vi "6 Cyl Diesel with 1 VR Crank + 2 Hall Cams + Knock.vi"() -> ()   [LabVIEW 2013]
uses:
  Version Token.ctl
  APU/Settings.ctl
  APU/Input.ctl
  APU/Output.ctl
  Analog Replay/Settings.ctl
  Analog Replay/Input.ctl
  Analog Replay/Load Input.ctl
  Digital Pattern Generation/Load Input.ctl
  Digital Pattern Generation/Settings.ctl
  Digital Pattern Generation/Input.ctl
  ECU Event/Timing/Measure Output.ctl
  ECU Event/Timing/Measure Settings.ctl
  ECU Event/Timing/Capture Output.ctl
  Knock Sensor/Generate Input.ctl
  Knock Sensor/Cylinder Input.ctl
  Knock Sensor/Cylinder Settings.ctl
  Knock Sensor/Generate Settings.ctl
  APU/Shared Settings.ctl
  <vilib>/Platform/TimedLoop/XDataNode/timing_clust.ctl
  <vilib>/Platform/TimedLoop/XDataNode/nitl_modes.ctl
  <vilib>/Platform/TimedLoop/XDataNode/wakeup.ctl
  ECU Event/Timing/Capture Settings.ctl
  <vilib>/rvi/DataTransferAndStorage/Container/Common/niFpgaContainerGetUniqueNameForEmu.vi
  <vilib>/rvi/DataTransferAndStorage/Container/Common/niFpgaContainerSetEmuInfo.vi
  <vilib>/rvi/eio/common/nirviEmuReportErrorAndStop.vi
  <vilib>/rvi/Emulation/niFpgaSctlEmulationGetInTimedLoop.vi
  <vilib>/rvi/Emulation/niFpgaEmulationReportErrorSimple.vi
  <vilib>/rvi/Emulation/niFpgaGetClockAttributes.vi
  <vilib>/rvi/Emulation/niFpgaCriticalErrorInLSC.vi
  <vilib>/rvi/eio/common/nirviEmuTemplateMethod_errors.vi
  ECU Event/Timing/Measure Events (40MHz).vi
  <vilib>/Platform/TimedLoop/XDataNode/XDataNode.xnode
  <vilib>/rvi/LocalResourceManager/LocalResourceManager.xnode
  <vilib>/eio/EIONode/EIONode.xnode
  <vilib>/Platform/TimedLoop/XDataNode/XDNodeRunTimeDep.lvlib
  APU/APU.lvlib
  Analog Replay/Analog Replay.lvlib
  Digital Pattern Generation/Digital Pattern Generation.lvlib
  ECU Event/Timing/ECU Event Timing.lvlib
  Knock Sensor/Knock Sensor.lvlib
  Engine Simulation Toolkit.lvlib
panel:
  in  "shared settings.apu 1":T1 {"cycle start" format="%#.15g"}
  in  "go.apu 1":bool
  in  "settings.Knock AO 2.Cylinder 5":T2
  in  "settings.Knock AO 2.Cylinder 6":T2
  in  "input.Knock AO 2.Cylinder 5":T3={"probability compare"=65535, "high freq scaler"=0.0, "trigger position"=0}
  in  "input.Knock AO 2.Cylinder 6":T3={"probability compare"=65535, "high freq scaler"=0.0, "trigger position"=0}
  in  "settings.Knock AO 2":T4
  in  "settings.Knock AO 2.Cylinder 1":T2
  in  "settings.Knock AO 2.Cylinder 2":T2
  in  "settings.Knock AO 2.Cylinder 3":T2
  in  "settings.Knock AO 2.Cylinder 4":T2
  in  "input.Knock AO 2.Cylinder 1":T3={"probability compare"=65535, "high freq scaler"=0.0, "trigger position"=0}
  in  "input.Knock AO 2.Cylinder 2":T3={"probability compare"=65535, "high freq scaler"=0.0, "trigger position"=0}
  in  "input.Knock AO 2.Cylinder 3":T3={"probability compare"=65535, "high freq scaler"=0.0, "trigger position"=0}
  in  "input.Knock AO 2.Cylinder 4":T3={"probability compare"=65535, "high freq scaler"=0.0, "trigger position"=0}
  in  "input.Knock AO 2":T5
  out "capture.Injection DIO 15.Event 4":T6
  out "capture.Injection DIO 15.Event 3":T6
  out "capture.Injection DIO 15.Event 2":T6
  out "capture.Injection DIO 14.Event 4":T6
  out "capture.Injection DIO 14.Event 3":T6
  out "capture.Injection DIO 14.Event 2":T6
  out "capture.Injection DIO 13.Event 4":T6
  out "capture.Injection DIO 13.Event 3":T6
  out "capture.Injection DIO 13.Event 2":T6
  out "capture.Injection DIO 12.Event 4":T6
  out "capture.Injection DIO 12.Event 3":T6
  out "capture.Injection DIO 12.Event 2":T6
  out "capture.Injection DIO 11.Event 4":T6
  out "capture.Injection DIO 11.Event 3":T6
  out "capture.Injection DIO 11.Event 2":T6
  out "capture.Injection DIO 10.Event 4":T6
  out "capture.Injection DIO 10.Event 3":T6
  out "capture.Injection DIO 10.Event 2":T6
  out "capture.Injection DIO 10.Event 1":T6
  out "capture.Injection DIO 11.Event 1":T6
  out "capture.Injection DIO 12.Event 1":T6
  out "capture.Injection DIO 13.Event 1":T6
  out "capture.Injection DIO 14.Event 1":T6
  out "capture.Injection DIO 15.Event 1":T6
  in  "settings.Injection DIO 10":T7
  in  "settings.Injection DIO 11":T7
  in  "settings.Injection DIO 12":T7
  in  "settings.Injection DIO 13":T7
  in  "settings.Injection DIO 14":T7
  in  "settings.Injection DIO 15":T7
  out "status.Injection DIO 10":T8
  out "status.Injection DIO 11":T8
  out "status.Injection DIO 12":T8
  out "status.Injection DIO 13":T8
  out "status.Injection DIO 14":T8
  out "status.Injection DIO 15":T8
  in  "load input.Cam2 DIO 1":T9
  in  "input.Cam1 DIO 0":T10
  in  "settings.Cam1 DIO 0":T11
  in  "input.Cam2 DIO 1":T10
  in  "settings.Cam2 DIO 1":T11
  in  "load input.Cam1 DIO 0":T9
  in  "load input.Crank AO 0":T12={"Data"=[0, 0, 0, 0, 0, 0, 0, 0, 0, 0, 0, 0, 0, 0, 0, 0], "LoadOffset"=0, "Done"=FALSE} caption="input"
  in  "input.Crank AO 0":T13 caption="input"
  in  "settings.Crank AO 0":T14 caption="settings"
  out "output.apu 1":T15 caption="output"
  in  "input.apu 1":T16={"desired speed"=0.0, "reset"=TRUE} caption="input"
  in  "settings.apu 1":T17 caption="settings"
  in  "est.version":T18
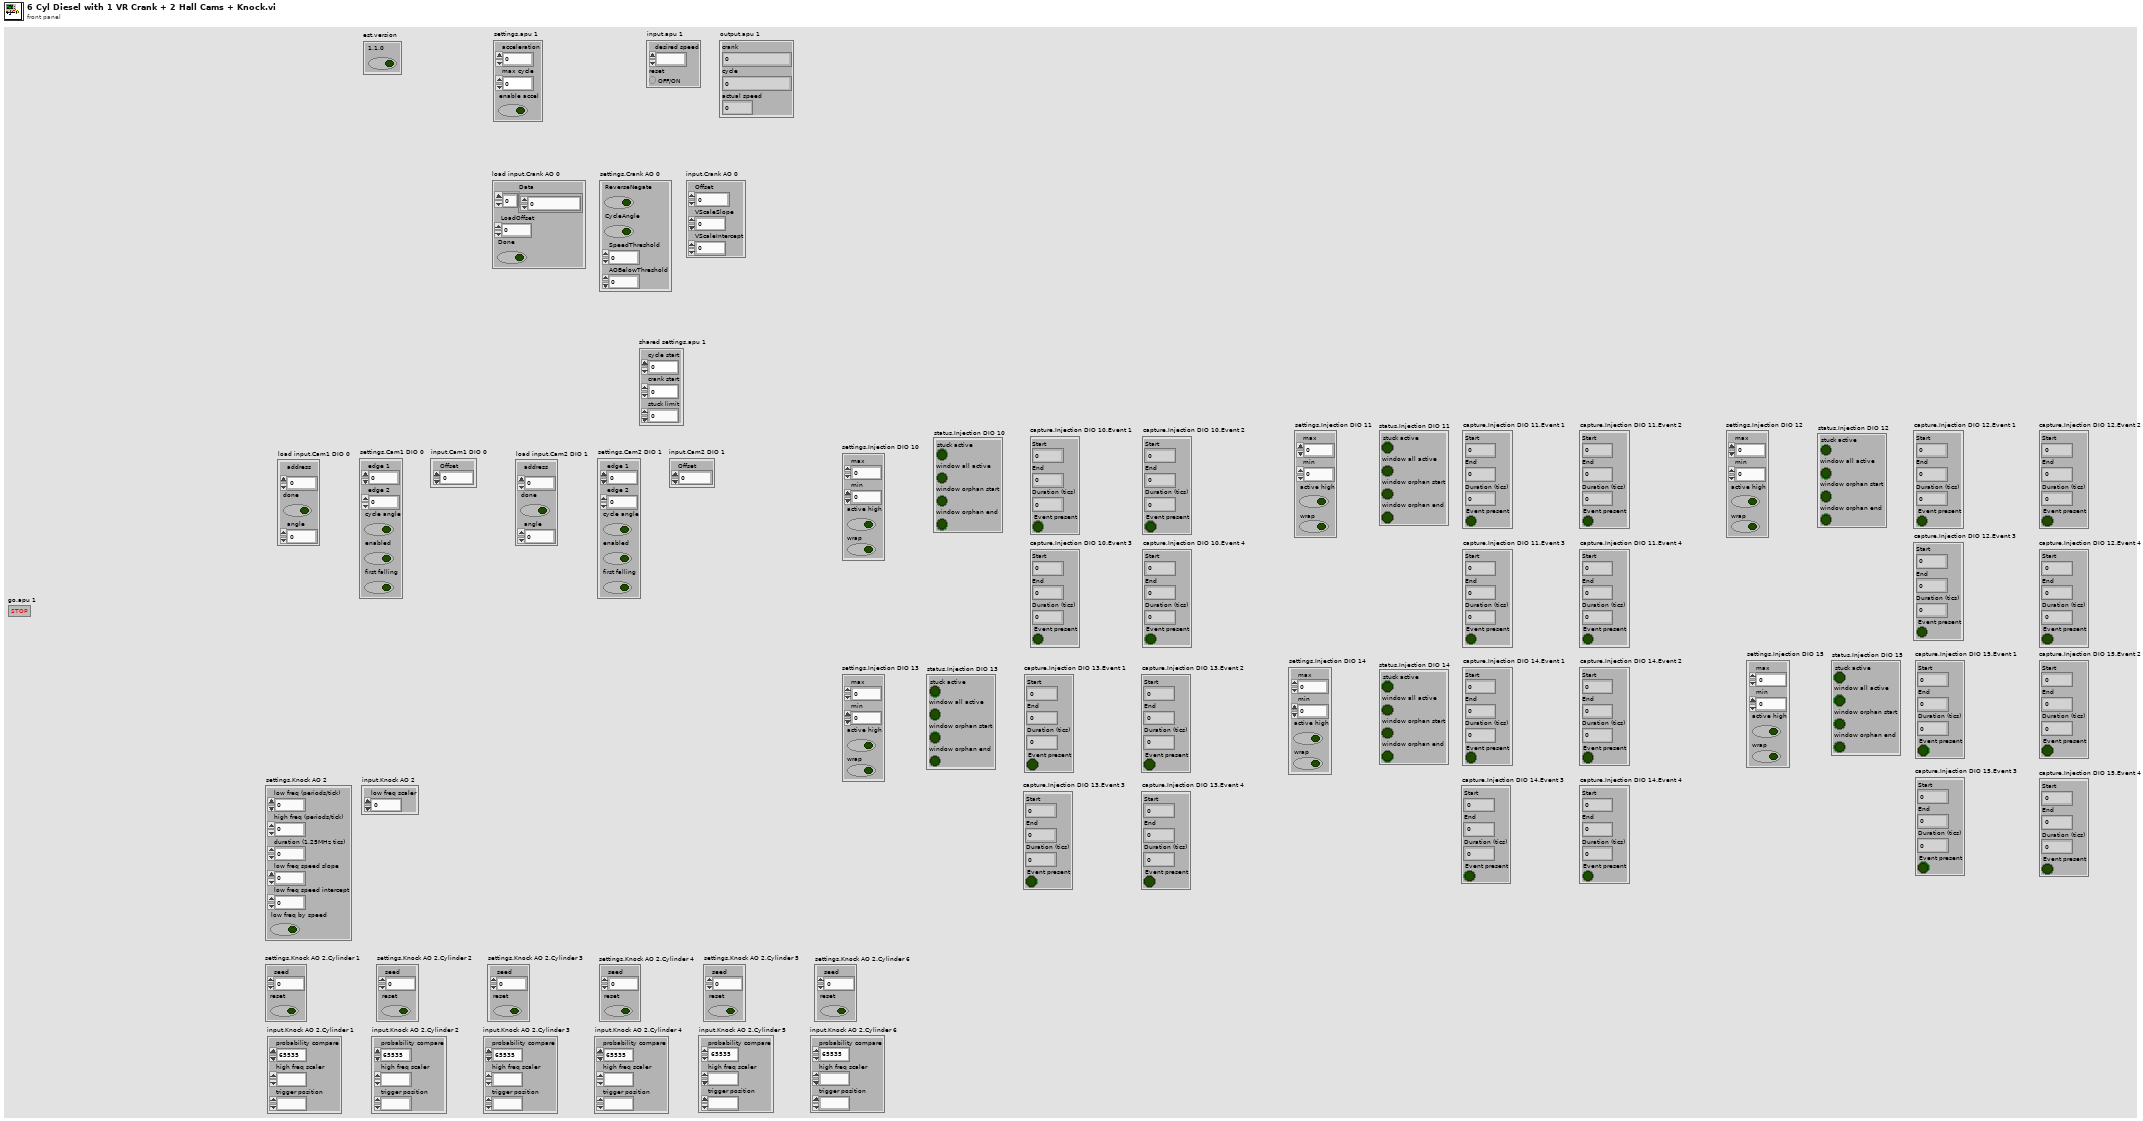
[diagram p1: front panel]
types:
  T1 = typedef "Engine Simulation Toolkit.lvlib/APU.lvlib/Shared Settings.ctl" = cluster{"cycle start":fxp<+,2,2>, "crank start":u16, "stuck limit":fxp<+,18,18>}
  T2 = typedef "Engine Simulation Toolkit.lvlib/Knock Sensor.lvlib/Cylinder Settings.ctl" = cluster{"seed":u16, "reset":bool}
  T3 = typedef "Engine Simulation Toolkit.lvlib/Knock Sensor.lvlib/Cylinder Input.ctl" = cluster{"probability compare":u16, "high freq scaler":fxp<+,10,0>, "trigger position":u16}
  T4 = typedef "Engine Simulation Toolkit.lvlib/Knock Sensor.lvlib/Generate Settings.ctl" = cluster{"low freq (periods/tick)":fxp<+,32,0>, "high freq (periods/tick)":fxp<+,32,0>, "duration (1.25MHz tics)":fxp<+,18,18>, "low freq speed slope":fxp<+,16,-3>, "low freq speed intercept":fxp<+,10,-10>, "low freq by speed":bool}
  T5 = typedef "Engine Simulation Toolkit.lvlib/Knock Sensor.lvlib/Generate Input.ctl" = cluster{"low freq scaler":fxp<+,10,0>}
  T6 = typedef "Engine Simulation Toolkit.lvlib/ECU Event Timing.lvlib/Capture Output.ctl" = cluster{"Start":u16, "End":u16, "Duration (tics)":fxp<+,18,18>, "Event present":bool}
  T7 = typedef "Engine Simulation Toolkit.lvlib/ECU Event Timing.lvlib/Measure Settings.ctl" = cluster{"max":u16, "min":u16, "active high":bool, "wrap":bool}
  T8 = typedef "Engine Simulation Toolkit.lvlib/ECU Event Timing.lvlib/Measure Output.ctl" = cluster{"stuck active":bool, "window all active":bool, "window orphan start":bool, "window orphan end":bool}
  T9 = typedef "Engine Simulation Toolkit.lvlib/Digital Pattern Generation.lvlib/Load Input.ctl" = cluster{"address":fxp<+,11,11>, "done":bool, "angle":u16}
  T10 = typedef "Engine Simulation Toolkit.lvlib/Digital Pattern Generation.lvlib/Input.ctl" = cluster{"Offset":i16}
  T11 = typedef "Engine Simulation Toolkit.lvlib/Digital Pattern Generation.lvlib/Settings.ctl" = cluster{"edge 1":u16, "edge 2":u16, "cycle angle":bool, "enabled":bool, "first falling":bool}
  T12 = typedef "Engine Simulation Toolkit.lvlib/Analog Replay.lvlib/Load Input.ctl" = cluster{"Data":i16[], "LoadOffset":u16, "Done":bool}
  T13 = typedef "Engine Simulation Toolkit.lvlib/Analog Replay.lvlib/Input.ctl" = cluster{"Offset":i16, "VScaleSlope":fxp<+,18,6>, "VScaleIntercept":fxp<+/-,18,3>}
  T14 = typedef "Engine Simulation Toolkit.lvlib/Analog Replay.lvlib/Settings.ctl" = cluster{"ReverseNegate":bool, "CycleAngle":bool, "SpeedThreshold":fxp<+/-,23,2>, "AOBelowThreshold":i16}
  T15 = typedef "Engine Simulation Toolkit.lvlib/APU.lvlib/Output.ctl" = cluster{"crank":u16, "cycle":u16, "actual speed":fxp<+/-,23,2>}
  T16 = typedef "Engine Simulation Toolkit.lvlib/APU.lvlib/Input.ctl" = cluster{"desired speed":fxp<+/-,23,2>, "reset":bool}
  T17 = typedef "Engine Simulation Toolkit.lvlib/APU.lvlib/Settings.ctl" = cluster{"acceleration":fxp<+,18,-20>, "max cycle":fxp<+,2,2>, "enable accel":bool}
  T18 = typedef "Engine Simulation Toolkit.lvlib/Version Token.ctl" = cluster{"1.1.0":bool}
  T19 = typedef "XDNodeRunTimeDep.lvlib/timing_clust.ctl" = cluster{"Expected End [f-1]":u64, "Actual End [f-1]":u64, "Finished Late? [f-1]":bool, "Expected End [i-1]":u64, "Actual End [i-1]":u64, "Finished Late? [i-1]":bool, "Expected Start [i]":u64, "Actual Start [i]":u64, "Expected Start [f]":u64, "Actual Start [f]":u64, "Source Name":string, "Structure Name":string, "Period":i64, "Deadline":i64, "Offset":i64, "Start":i64, "Priority":i32, "Timeout":i32, "Mode":T20, "Wakeup Reason":T21, "Error":errorcluster, "Source Type":string, "Secondary Source Type":string, "Global End Time":u64, "Global Start Time":u64, "Frame Duration":u64, "Iteration Duration":u64, "Assigned CPU":i32, "I/O Scan Engine Mode":u32}
  T20 = typedef "XDNodeRunTimeDep.lvlib/nitl_modes.ctl" = enum32{"No Change", "Process missed periods, maintain original phase", "Discard missed periods, maintain original phase", "Process missed periods, ignore original phase", "Discard missed periods, ignore original phase"}
  T21 = typedef "XDNodeRunTimeDep.lvlib/wakeup.ctl" = enum32{"Normal", "Aborted", "Asynchronous wakeup", "Timing source error", "Timed loop error", "Timeout"}
  T22 = typedef "Engine Simulation Toolkit.lvlib/APU.lvlib/Register Bus.ctl" = cluster{"Speed":refnum<k21>, "Crank Angle":refnum<k21>, "Cycle Angle":refnum<k21>, "Crank Count":refnum<k21>, "Cycle Count":refnum<k21>, "1.25 MHz Counter":refnum<k21>, "shared settings":T1}
  T23 = typedef "Engine Simulation Toolkit.lvlib/Digital Pattern Generation.lvlib/Load Data.ctl" = cluster{"max address":fxp<+,11,11>, "memory":refnum<k21>}
  T24 = typedef "Engine Simulation Toolkit.lvlib/Knock Sensor.lvlib/Triggered Cylinder Data.ctl" = cluster{"trigger knock":bool, "high freq scaler":fxp<+,10,0>}
  T25 = typedef "Engine Simulation Toolkit.lvlib/ECU Event Timing.lvlib/Capture Settings.ctl" = u8
  T26 = typedef "Engine Simulation Toolkit.lvlib/ECU Event Timing.lvlib/Measured Data.ctl" = cluster{"start":u16, "end":u16, "duration (tics)":fxp<+,18,18>, "window end":bool, "window begin":bool, "pulse end":bool, "pulse #":u8}
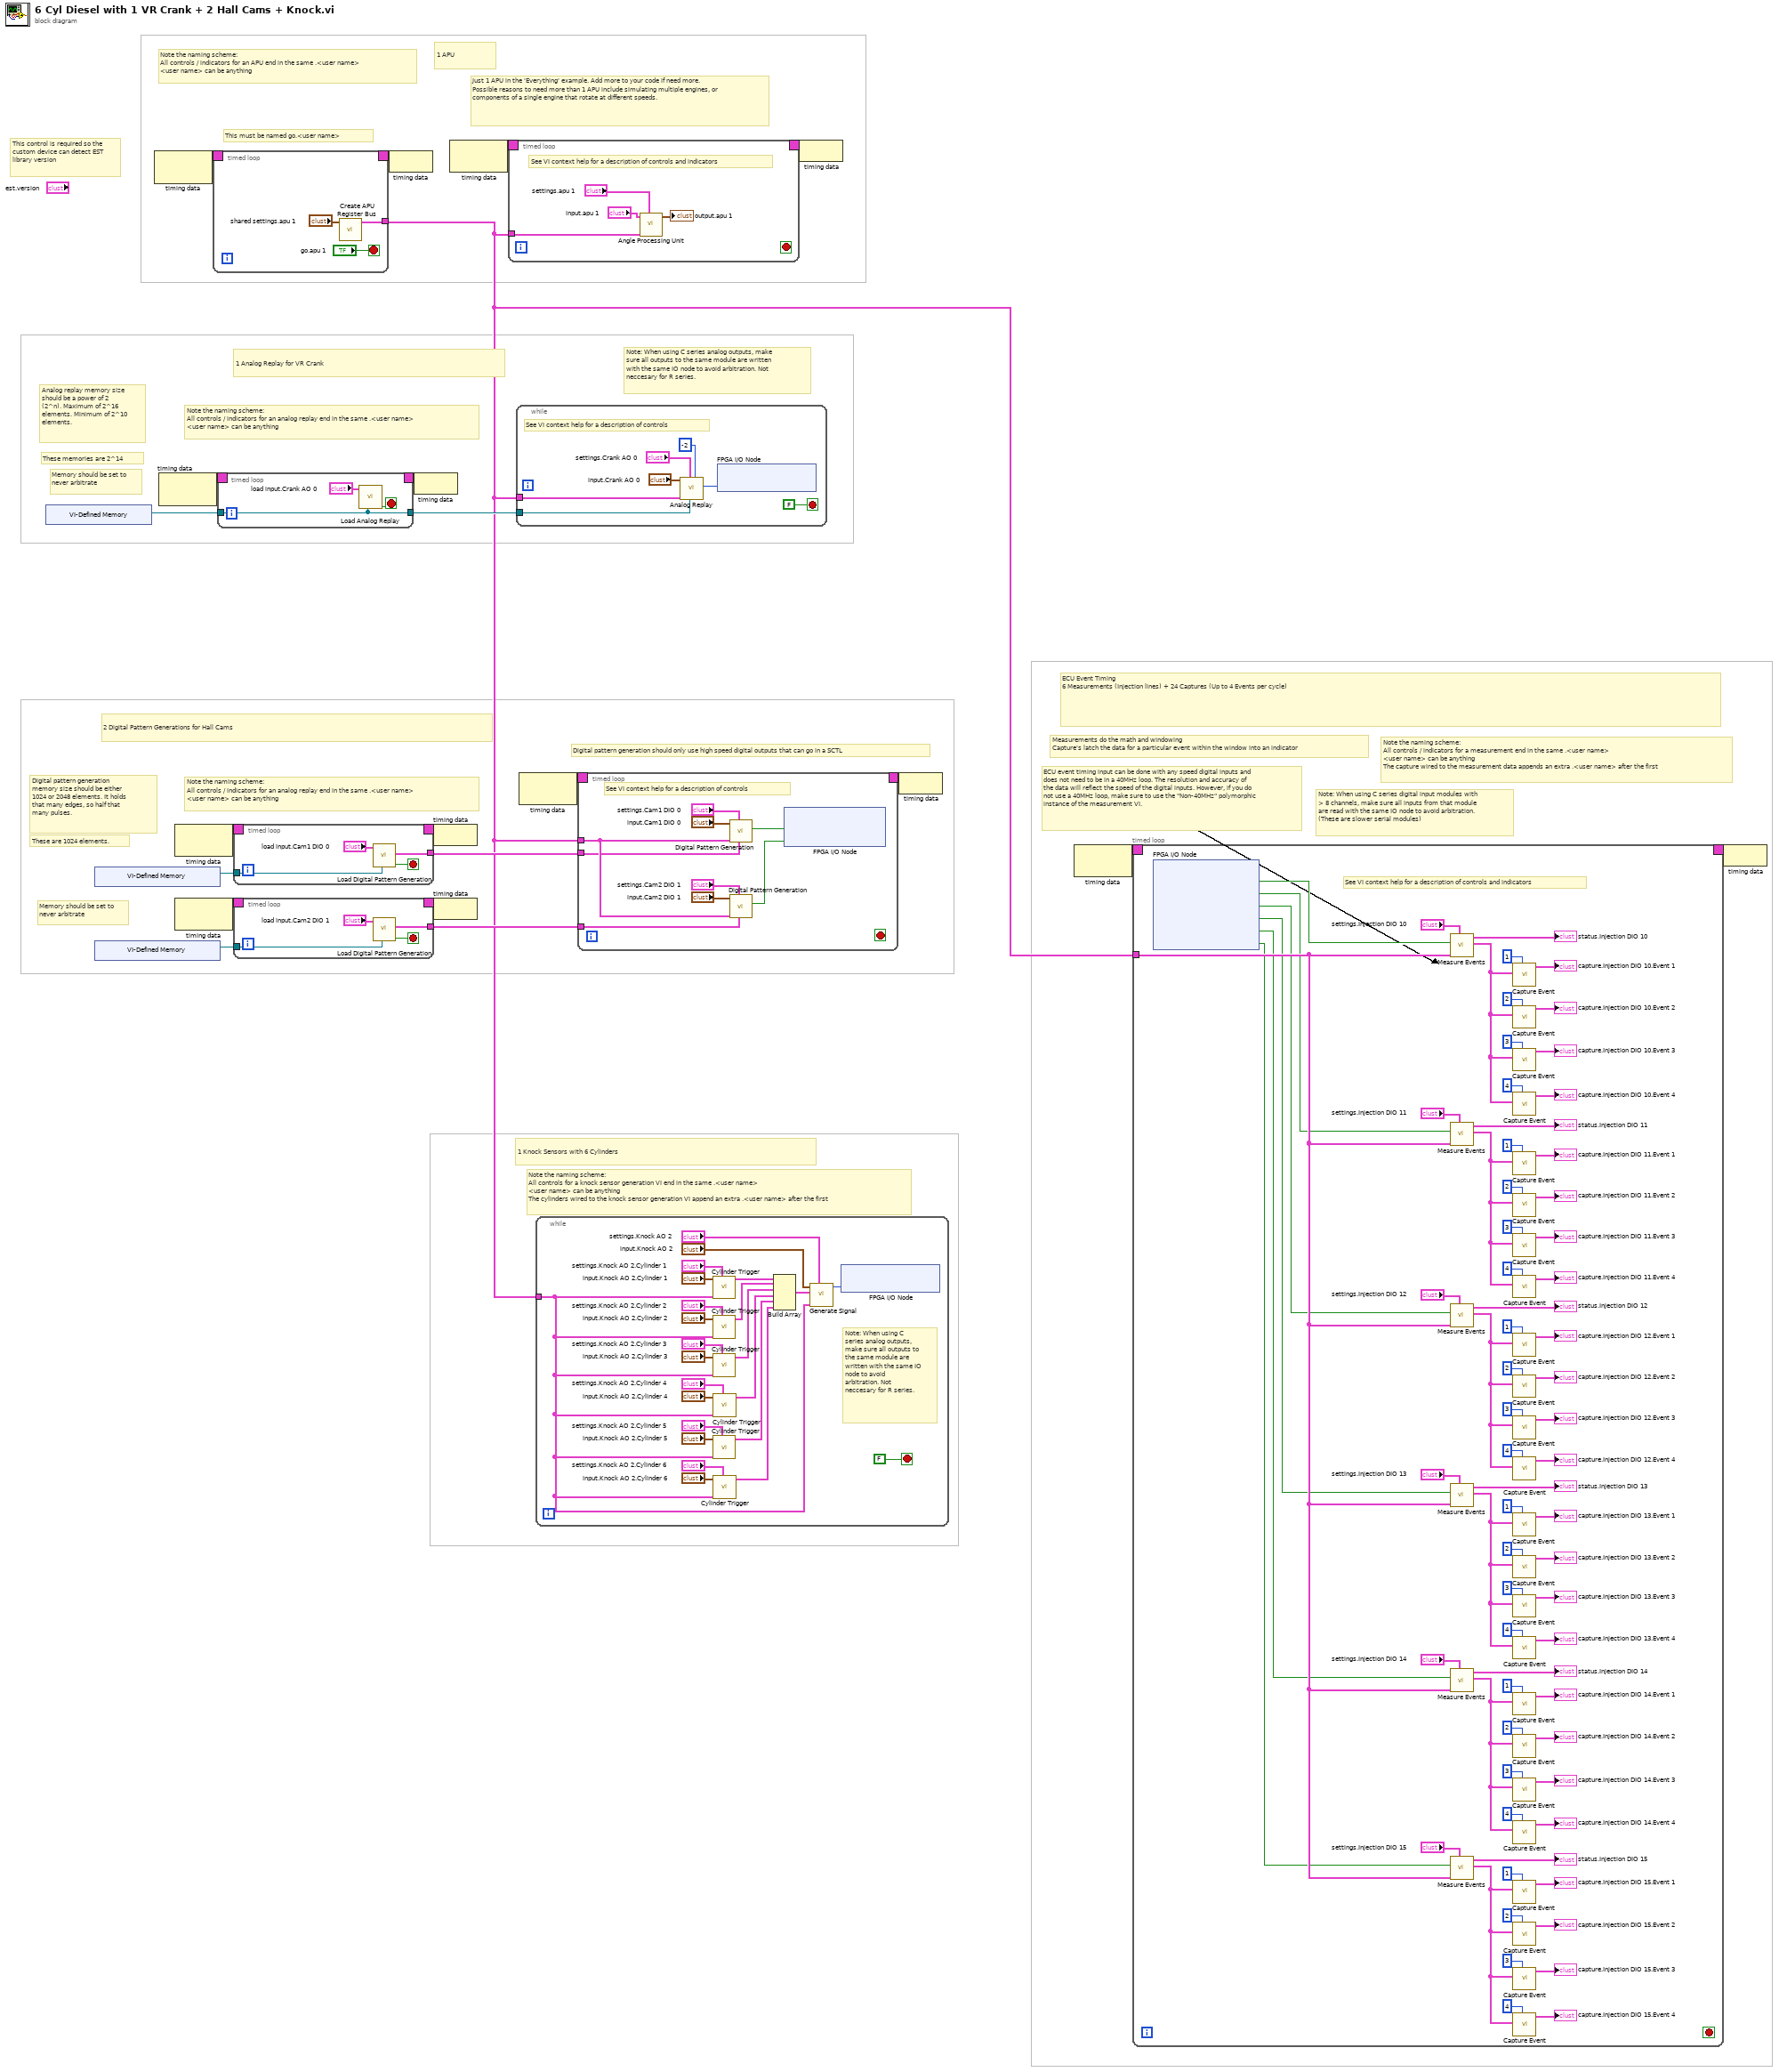
[diagram p0: block diagram]
diagram:
  # "This must be named go.<user name>"
  # "Memory should be set to never arbitrate"
  # "Memory should be set to never arbitrate"
  # "Note the naming scheme: \nAll controls for a knock sensor generation VI end in the same .<user name>\n<user name> can be anything\nThe cylinders wired to the knock sensor generation VI append an extra .<user name> after the first"
  # "1 Knock Sensors with 6 Cylinders"
  # "Measurements do the math and windowing\nCapture's latch the data for a particular event within the window into an indicator"
  # "ECU Event Timing\n6 Measurements (Injection lines) + 24 Captures (Up to 4 Events per cycle)"
  # "Note the naming scheme: \nAll controls / indicators for a measurement end in the same .<user name>\n<user name> can be anything\nThe capture wired to the measurement data appends an extra .<user name> after the first"
  # "Note: When using C series digital input modules with > 8 channels, make sure all inputs from that module are read with the same IO node to avoid arbitration. (These are slower serial modules)"
  # "ECU event timing input can be done with any speed digital inputs and does not need to be in a 40MHz loop. The resolution and accuracy of the data will reflect the speed of the digital inputs. However, if you do not use a 40MHz loop, make sure to use the \"Non-40MHz\" polymorphic instance of the measurement VI."
  # "Digital pattern generation should only use high speed digital outputs that can go in a SCTL"
  # "2 Digital Pattern Generations for Hall Cams"
  # "Note the naming scheme: \nAll controls / indicators for an analog replay end in the same .<user name>\n<user name> can be anything"
  # "These are 1024 elements."
  # "Digital pattern generation memory size should be either 1024 or 2048 elements. It holds that many edges, so half that many pulses."
  # "Note: When using C series analog outputs, make sure all outputs to the same module are written with the same IO node to avoid arbitration. Not neccesary for R series."
  # "1 Analog Replay for VR Crank"
  # "1 APU"
  # "These memories are 2^14"
  # "Note the naming scheme: \nAll controls / indicators for an APU end in the same .<user name>\n<user name> can be anything"
  # "Note the naming scheme: \nAll controls / indicators for an analog replay end in the same .<user name>\n<user name> can be anything"
  # "Analog replay memory size should be a power of 2 (2^n). Maximum of 2^16 elements. Minimum of 2^10 elements."
  # "Just 1 APU in the 'Everything' example. Add more to your code if need more. Possible reasons to need more than 1 APU include simulating multiple engines, or components of a single engine that rotate at different speeds."
  # "This control is required so the custom device can detect EST library version"
  n1 = xnode "VI-Defined Memory"() -> ("Memory Out"=w17:refnum<k21>)
  n2 = xnode "VI-Defined Memory"() -> ("Memory Out"=w11:refnum<k21>)
  n3 = xnode "VI-Defined Memory"() -> ("Memory Out"=w7:refnum<k21>)
  n4 = node-c288() -> (w3:T19)  [unwired: 1 in]
  n5 = node-c288() -> (w19:T19)  [unwired: 1 in]
  n6 = node-c288() -> (w15:T19)  [unwired: 1 in]
  n7 = node-c288() -> (w9:T19)  [unwired: 1 in]
  n8 = timed-loop {
    timing: w3 -> [_]
    timing-out: [_] -> w2
    tunnel: [w23] -> w1
    stop <- "go.apu 1" stop-if-true
    n9 = call "Create APU Register Bus.vi"("shared settings.<user name>"="shared settings.apu 1") -> ("register bus"=w23:T22)  [unwired: 10 in]
  }
  n10 = timed-loop {
    timing: w19 -> [_]
    timing-out: [_] -> w18
    tunnel: w17 -> [w27]
    tunnel: [w27] -> w16
    stop <- w28 stop-if-true
    n11 = call "Load Analog Replay.vi"("memory"=w27, "load input.<user name>"="load input.Crank AO 0") -> ("done"=w28:bool)  [unwired: 9 in]
  }
  n12 = timed-loop {
    timing: w15 -> [_]
    timing-out: [_] -> w14
    tunnel: w11 -> [w34]
    tunnel: [w33] -> w10
    stop <- w35 stop-if-true
    n13 = call "Load Digital Pattern Generation.vi"("memory"=w34, "load input.<user name>"="load input.Cam1 DIO 0") -> ("done"=w35:bool, "load data"=w33:T23)  [unwired: 8 in]
  }
  n14 = timed-loop {
    timing: w9 -> [_]
    timing-out: [_] -> w8
    tunnel: w7 -> [w40]
    tunnel: [w39] -> w6
    stop <- w41 stop-if-true
    n15 = call "Load Digital Pattern Generation.vi"("memory"=w40, "load input.<user name>"="load input.Cam2 DIO 1") -> ("done"=w41:bool, "load data"=w39:T23)  [unwired: 8 in]
  }
  n16 = node-c288(w2) -> ()
  n17 = node-c288(w18) -> ()
  n18 = node-c288(w14) -> ()
  n19 = node-c288(w8) -> ()
  n20 = node-c288() -> (w21:T19)  [unwired: 1 in]
  n21 = timed-loop {
    timing: w21 -> [_]
    timing-out: [_] -> w20
    tunnel: w1 -> [w44]
    stop <- _ stop-if-true
    # "See VI context help for a description of controls and indicators"
    n22 = call "Angle Processing Unit.vi"("settings.<user name>"="settings.apu 1", "register bus"=w44, "input.<user name>"="input.apu 1") -> ("output.<user name>"=→"output.apu 1":T15)  [unwired: 8 in]
  }
  n23 = while {
    tunnel: w16 -> [w56]
    tunnel: w1 -> [w50]
    stop <- FALSE stop-if-true
    # "See VI context help for a description of controls"
    n24 = call "Analog Replay.vi"("shift"=i8 -2, "memory"=w56, "settings.<user name>"="settings.Crank AO 0", "register bus"=w50, "input.<user name>"="input.Crank AO 0") -> ("analog value"=w51:i16)  [unwired: 6 in]
    n25 = xnode "FPGA I/O Node"("Connector0/AO0"=w51) -> ()  [unwired: 1 in, 1 out]
  }
  n26 = node-c288() -> (w13:T19)  [unwired: 1 in]
  n27 = while {
    tunnel: w1 -> [w57]
    stop <- FALSE stop-if-true
    # "Note: When using C series analog outputs, make sure all outputs to the same module are written with the same IO node to avoid arbitration. Not neccesary for R series."
    n28 = call "Cylinder Trigger.vi"("settings.<user name>"="settings.Knock AO 2.Cylinder 1", "register bus"=w57, "input.<user name>"="input.Knock AO 2.Cylinder 1") -> ("triggered knock data"=w80:T24)  [unwired: 8 in]
    n29 = call "Cylinder Trigger.vi"("settings.<user name>"="settings.Knock AO 2.Cylinder 2", "register bus"=w57, "input.<user name>"="input.Knock AO 2.Cylinder 2") -> ("triggered knock data"=w79:T24)  [unwired: 8 in]
    n30 = call "Cylinder Trigger.vi"("settings.<user name>"="settings.Knock AO 2.Cylinder 3", "register bus"=w57, "input.<user name>"="input.Knock AO 2.Cylinder 3") -> ("triggered knock data"=w78:T24)  [unwired: 8 in]
    n31 = call "Cylinder Trigger.vi"("settings.<user name>"="settings.Knock AO 2.Cylinder 5", "register bus"=w57, "input.<user name>"="input.Knock AO 2.Cylinder 5") -> ("triggered knock data"=w59:T24)  [unwired: 8 in]
    n32 = call "Cylinder Trigger.vi"("settings.<user name>"="settings.Knock AO 2.Cylinder 4", "register bus"=w57, "input.<user name>"="input.Knock AO 2.Cylinder 4") -> ("triggered knock data"=w77:T24)  [unwired: 8 in]
    n33 = call "Cylinder Trigger.vi"("settings.<user name>"="settings.Knock AO 2.Cylinder 6", "register bus"=w57, "input.<user name>"="input.Knock AO 2.Cylinder 6") -> ("triggered knock data"=w58:T24)  [unwired: 8 in]
    n34 = Build Array(w80, w79, w78, w77, w59, w58) -> (w76:T24[])
    n35 = call "Generate Signal.vi"("settings.<user name>"="settings.Knock AO 2", "register bus"=w57, "triggered knock data"=w76, "input.<user name>"="input.Knock AO 2") -> ("knock signal"=w64:i16)  [unwired: 7 in]
    n36 = xnode ("FPGA I/O Node")("Connector0/AO2"=w64) -> ()  [unwired: 1 in, 1 out]
  }
  n37 = timed-loop {
    tunnel: w1 -> [w83]
    timing: w13 -> [_]
    timing-out: [_] -> w12
    tunnel: w10 -> [w82]
    tunnel: w6 -> [w81]
    stop <- _ stop-if-true
    # "See VI context help for a description of controls"
    n38 = call "Digital Pattern Generation.vi"("load data"=w82, "settings.<user name>"="settings.Cam1 DIO 0", "register bus"=w83, "input.<user name>"="input.Cam1 DIO 0") -> ("digial output"=w86:bool)  [unwired: 7 in]
    n39 = call "Digital Pattern Generation.vi"("load data"=w81, "settings.<user name>"="settings.Cam2 DIO 1", "register bus"=w83, "input.<user name>"="input.Cam2 DIO 1") -> ("digial output"=w87:bool)  [unwired: 7 in]
    n40 = xnode "FPGA I/O Node"("Connector0/DIO0"=w86, "Connector0/DIO1"=w87) -> ()  [unwired: 2 in, 2 out]
  }
  n41 = node-c288(w20) -> ()
  n42 = node-c288(w12) -> ()
  n43 = node-c288() -> (w5:T19)  [unwired: 1 in]
  n44 = timed-loop {
    timing: w5 -> [_]
    timing-out: [_] -> w4
    tunnel: w1 -> [w158]
    stop <- _ stop-if-true
    # "See VI context help for a description of controls and indicators"
    n45 = xnode "FPGA I/O Node"() -> ("Connector0/DIO10"=w145:bool, "Connector0/DIO11"=w144:bool, "Connector0/DIO12"=w143:bool, "Connector0/DIO13"=w142:bool, "Connector0/DIO14"=w141:bool, "Connector0/DIO15"=w140:bool)  [unwired: 6 in, 6 out]
    n46 = call-poly "Measure Events.vi"("settings.<user name>"="settings.Injection DIO 10", "register bus"=w158, "event"=w145) -> ("measured data"=w127:T26, "status.<user name>"=→"status.Injection DIO 10":T8)  [unwired: 7 in]
    n47 = call-poly "Measure Events.vi"("settings.<user name>"="settings.Injection DIO 11", "register bus"=w158, "event"=w144) -> ("measured data"=w120:T26, "status.<user name>"=→"status.Injection DIO 11":T8)  [unwired: 7 in]
    n48 = call-poly "Measure Events.vi"("settings.<user name>"="settings.Injection DIO 12", "register bus"=w158, "event"=w143) -> ("measured data"=w113:T26, "status.<user name>"=→"status.Injection DIO 12":T8)  [unwired: 7 in]
    n49 = call-poly "Measure Events.vi"("settings.<user name>"="settings.Injection DIO 13", "register bus"=w158, "event"=w142) -> ("measured data"=w106:T26, "status.<user name>"=→"status.Injection DIO 13":T8)  [unwired: 7 in]
    n50 = call-poly "Measure Events.vi"("settings.<user name>"="settings.Injection DIO 14", "register bus"=w158, "event"=w141) -> ("measured data"=w99:T26, "status.<user name>"=→"status.Injection DIO 14":T8)  [unwired: 7 in]
    n51 = call-poly "Measure Events.vi"("settings.<user name>"="settings.Injection DIO 15", "register bus"=w158, "event"=w140) -> ("measured data"=w92:T26, "status.<user name>"=→"status.Injection DIO 15":T8)  [unwired: 7 in]
    n52 = call "Capture Event.vi"("event # to capture"=T25 1 ("Settings.spark 1 shot 1"), "measured data"=w127) -> ("capture.<user name>"=→"capture.Injection DIO 10.Event 1":T6)  [unwired: 9 in]
    n53 = call "Capture Event.vi"("event # to capture"=T25 2 ("Settings.spark 1 shot 1"), "measured data"=w127) -> ("capture.<user name>"=→"capture.Injection DIO 10.Event 2":T6)  [unwired: 9 in]
    n54 = call "Capture Event.vi"("event # to capture"=T25 3 ("Settings.spark 1 shot 1"), "measured data"=w127) -> ("capture.<user name>"=→"capture.Injection DIO 10.Event 3":T6)  [unwired: 9 in]
    n55 = call "Capture Event.vi"("event # to capture"=T25 4 ("Settings.spark 1 shot 1"), "measured data"=w127) -> ("capture.<user name>"=→"capture.Injection DIO 10.Event 4":T6)  [unwired: 9 in]
    n56 = call "Capture Event.vi"("event # to capture"=T25 1 ("Settings.spark 2 shot 1"), "measured data"=w120) -> ("capture.<user name>"=→"capture.Injection DIO 11.Event 1":T6)  [unwired: 9 in]
    n57 = call "Capture Event.vi"("event # to capture"=T25 2 ("Settings.spark 2 shot 1"), "measured data"=w120) -> ("capture.<user name>"=→"capture.Injection DIO 11.Event 2":T6)  [unwired: 9 in]
    n58 = call "Capture Event.vi"("event # to capture"=T25 3 ("Settings.spark 2 shot 1"), "measured data"=w120) -> ("capture.<user name>"=→"capture.Injection DIO 11.Event 3":T6)  [unwired: 9 in]
    n59 = call "Capture Event.vi"("event # to capture"=T25 4 ("Settings.spark 2 shot 1"), "measured data"=w120) -> ("capture.<user name>"=→"capture.Injection DIO 11.Event 4":T6)  [unwired: 9 in]
    n60 = call "Capture Event.vi"("event # to capture"=T25 1 ("Settings.spark 3 shot 1"), "measured data"=w113) -> ("capture.<user name>"=→"capture.Injection DIO 12.Event 1":T6)  [unwired: 9 in]
    n61 = call "Capture Event.vi"("event # to capture"=T25 2 ("Settings.spark 3 shot 1"), "measured data"=w113) -> ("capture.<user name>"=→"capture.Injection DIO 12.Event 2":T6)  [unwired: 9 in]
    n62 = call "Capture Event.vi"("event # to capture"=T25 3 ("Settings.spark 3 shot 1"), "measured data"=w113) -> ("capture.<user name>"=→"capture.Injection DIO 12.Event 3":T6)  [unwired: 9 in]
    n63 = call "Capture Event.vi"("event # to capture"=T25 4 ("Settings.spark 3 shot 1"), "measured data"=w113) -> ("capture.<user name>"=→"capture.Injection DIO 12.Event 4":T6)  [unwired: 9 in]
    n64 = call "Capture Event.vi"("event # to capture"=T25 1 ("Settings.spark 4 shot 1"), "measured data"=w106) -> ("capture.<user name>"=→"capture.Injection DIO 13.Event 1":T6)  [unwired: 9 in]
    n65 = call "Capture Event.vi"("event # to capture"=T25 2 ("Settings.spark 4 shot 1"), "measured data"=w106) -> ("capture.<user name>"=→"capture.Injection DIO 13.Event 2":T6)  [unwired: 9 in]
    n66 = call "Capture Event.vi"("event # to capture"=T25 3 ("Settings.spark 4 shot 1"), "measured data"=w106) -> ("capture.<user name>"=→"capture.Injection DIO 13.Event 3":T6)  [unwired: 9 in]
    n67 = call "Capture Event.vi"("event # to capture"=T25 4 ("Settings.spark 4 shot 1"), "measured data"=w106) -> ("capture.<user name>"=→"capture.Injection DIO 13.Event 4":T6)  [unwired: 9 in]
    n68 = call "Capture Event.vi"("event # to capture"=T25 1 ("Settings.spark 5 shot 1"), "measured data"=w99) -> ("capture.<user name>"=→"capture.Injection DIO 14.Event 1":T6)  [unwired: 9 in]
    n69 = call "Capture Event.vi"("event # to capture"=T25 2 ("Settings.spark 5 shot 1"), "measured data"=w99) -> ("capture.<user name>"=→"capture.Injection DIO 14.Event 2":T6)  [unwired: 9 in]
    n70 = call "Capture Event.vi"("event # to capture"=T25 3 ("Settings.spark 5 shot 1"), "measured data"=w99) -> ("capture.<user name>"=→"capture.Injection DIO 14.Event 3":T6)  [unwired: 9 in]
    n71 = call "Capture Event.vi"("event # to capture"=T25 4 ("Settings.spark 5 shot 1"), "measured data"=w99) -> ("capture.<user name>"=→"capture.Injection DIO 14.Event 4":T6)  [unwired: 9 in]
    n72 = call "Capture Event.vi"("event # to capture"=T25 1 ("Settings.spark 6 shot 1"), "measured data"=w92) -> ("capture.<user name>"=→"capture.Injection DIO 15.Event 1":T6)  [unwired: 9 in]
    n73 = call "Capture Event.vi"("event # to capture"=T25 2 ("Settings.spark 6 shot 1"), "measured data"=w92) -> ("capture.<user name>"=→"capture.Injection DIO 15.Event 2":T6)  [unwired: 9 in]
    n74 = call "Capture Event.vi"("event # to capture"=T25 3 ("Settings.spark 6 shot 1"), "measured data"=w92) -> ("capture.<user name>"=→"capture.Injection DIO 15.Event 3":T6)  [unwired: 9 in]
    n75 = call "Capture Event.vi"("event # to capture"=T25 4 ("Settings.spark 6 shot 1"), "measured data"=w92) -> ("capture.<user name>"=→"capture.Injection DIO 15.Event 4":T6)  [unwired: 9 in]
  }
  n76 = node-c288(w4) -> ()
